vi "SENS_CORR_CCH_PAR_M.vi"(0 "VISA IN":refnum<visa-resource-name>, 1 "Measurement":string, 5 "error in":errorcluster, 7 "Channel":i32=1) -> (14 "VISA Out":refnum<visa-resource-name>, 19 "error out":errorcluster)   [LabVIEW 2018, in "PNA-X.lvlib"]
doc: "SENSe<cnum>:CORRection:CCHeck:PARameter <Mname> \n1625\n\n(Read-Write) Specifies an existing measurement to be used for the Confidence Check. \nParameters \n<cnum> Any existing channel number. If unspecified, value is set to 1 \n<Mname> Name of the measurement you are selecting for the confidence check. The \nmeasurement must already exist. \nExamples SENS:CORR:CCH:PAR 'TEST' \n'selects the measurement \"test\" on channel 1 for the confidence \ncheck \nsense2:correction:ccheck:parameter 'test' \n'selects the measurement \"test\" on channel 2 for the confidence \ncheck \nQuery Syntax SENSe<cnum>:CORRection:CCHeck:PARameter? \nReturns the name of the selected measurement on channel <cnum>. \nReturn Type String \nDefault Not applicable"
uses:
  PNA-X.lvlib
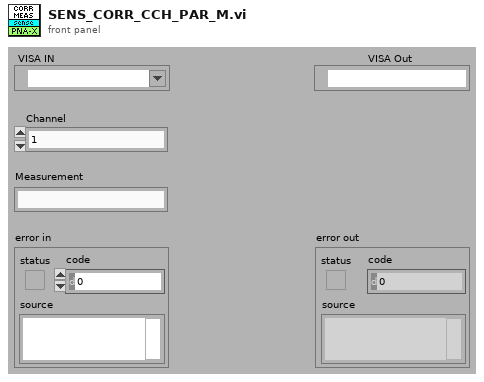
[diagram p1: front panel]
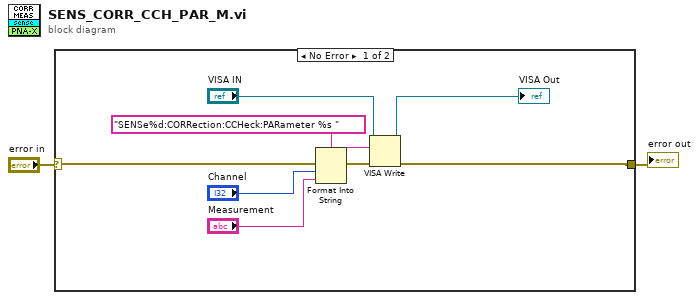
[diagram p0: block diagram]
diagram:
  n1 = case shown="No Error" "error in" {
    selector: "error in" -> [w11 w12]
    tunnel: [w6 w12] -> w1
    frame No Error {
      n2 = Format Into String(format string="SENSe%d:CORRection:CCHeck:PARameter %s " ("Cmdline"), error in=w11, "Channel", "Measurement") -> (resulting string=w9:string, error out=w10:errorcluster)  [unwired: 1 in]
      n3 = VISA Write(VISA resource name="VISA IN", write buffer=w9, error in (no error)=w10) -> (VISA resource name out=→"VISA Out":refnum<visa-resource-name>, error out=w6:errorcluster)  [unwired: 1 out]
    }
    frame Error {
    }
  }
  "error out" <- w1
